vi "Register_Publisher.vi"(11 "Baxter":T3={"topic port"=59814, "Node"="/labview", "topic"="/robot/head/command_head_nod", "type"="std_msgs/Bool", "node port"=7000, "error "={"status"=FALSE, "code"=0, "source"=""}, "Direction"=enum."Publisher", "APIs"=[]}) -> (0 "error out":errorcluster, 2 "connection ID out":refnum<k5>, 3 "Status":T1(ring), 5 "Subscribers":T2(array[cluster]))   [LabVIEW 2013]
doc: "Template server that runs individual ros topics, services, etc. This is cloned for each topic being run."
uses:
  ROS/Code/SubVIs/_ROSControl.ctl
  ROS/Code/SubVIs/_ROSDirection.ctl
  ROS/Code/_ROSDefinition.vi
panel:
  out "tcp":bool
  out "xml":bool
  out "time":u32
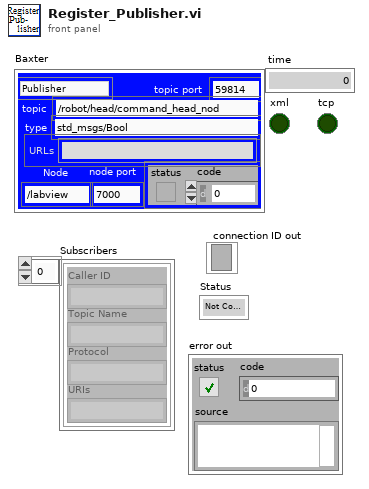
[diagram p1: front panel]
types:
  T1 = enum16{"Not Connected", "Registered", "Connected"}
  T2 = cluster{"Caller ID":string, "Topic Name":string, "Protocol":string, "URIs":string}[]
  T3 = typedef "_ROSControl.ctl" = cluster{"topic port":u16, "Node":string, "topic":string, "type":string, "node port":u32, "error ":errorcluster, "Direction":T4, "APIs":string[]}
  T4 = typedef "_ROSDirection.ctl" = enum16{"Node", "Publisher", "Subscriber", "Service Client"}
  T5 = cluster{"Code":i32, "Status Message":string, "APIs":string[]}
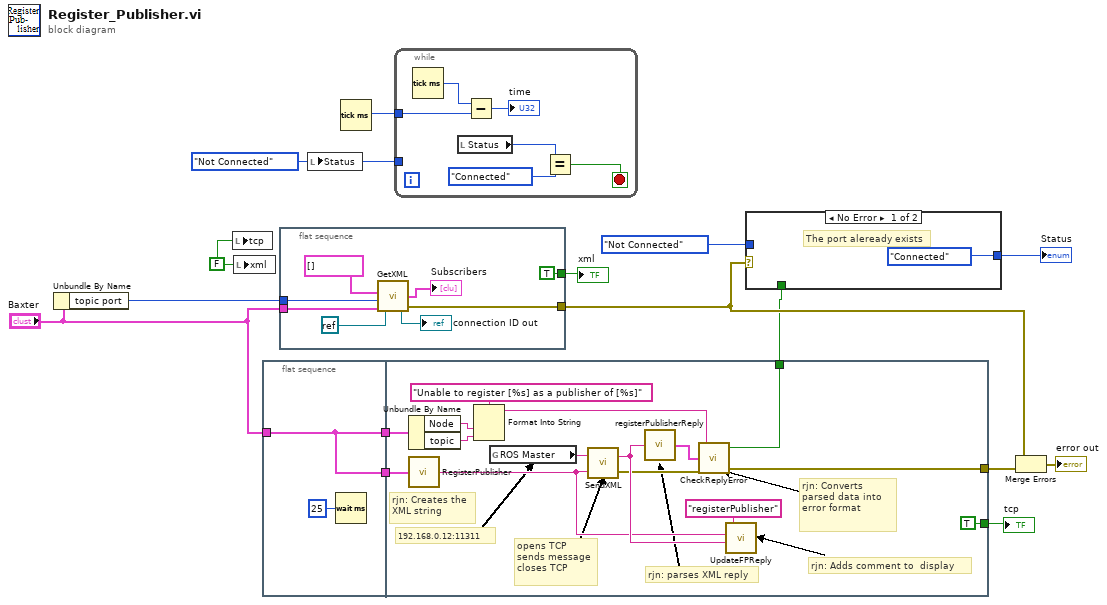
[diagram p0: block diagram]
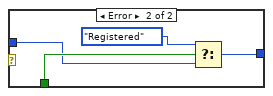
[diagram p2: hidden frame]
diagram:
  w1 = FALSE ("xml")
  w4 = T1."Not Connected" ("Status")
  n1 = Unbundle By Name("Baxter") -> ("topic port"=w15:u16)
  n2 = local write "tcp"(w1) -> ()
  n3 = local write "xml"(w1) -> ()
  n4 = flat-sequence {
    tunnel: "Baxter" -> [w16]
    tunnel: [w16] -> w13
    tunnel: [w16] -> w12
    tunnel: [w22] -> w9
    tunnel: [w20] -> w10
    tunnel: w13 -> [w21]
    tunnel: w12 -> [w19]
    tunnel: [TRUE] -> w2
    frame #0 {
      n5 = Wait (ms)(milliseconds to wait=u32 25) -> ()  [unwired: 1 out]
    }
    frame #1 {
      # "rjn: Adds comment to  display"
      # "rjn: Converts parsed data into\nerror format"
      # "rjn: parses XML reply"
      # "192.168.0.12:11311"
      # "opens TCP\nsends message\ncloses TCP"
      # "rjn: Creates the \nXML string"
      n6 = Unbundle By Name(w21) -> ("Node"=w28:string, "topic"=w27:string)
      n7 = call "RegisterPublisher.vi"("ROS"=w19) -> ("XML"=w26:string)
      n8 = Format Into String(format string="Unable to register [%s] as a publisher of [%s]", w28, w27) -> (resulting string=w24:string)  [unwired: 2 in, 1 out]
      n9 = global read "_ROSDefinition.vi" "ROS Master"() -> (w32:string)
      n10 = call "SendXML.vi"("Send"=w26, "URI in"=w32) -> ("error out"=w23:errorcluster, "Reply"=w31:string)
      n11 = call "registerPublisherReply.vi"("Response"=w31) -> ("Response"=w25:T5)
      n12 = call "CheckReplyError.vi"("error in"=w23, "Response"=w25, "Error String"=w24) -> ("error out"=w20:errorcluster, "Registered?"=w22:bool)  [unwired: 1 out]
      n13 = call "UpdateFPReply.vi"("Reply"=w31, "Sent"=w26, "method"="registerPublisher") -> ()  [unwired: 3 in]
    }
  }
  n14 = flat-sequence {
    tunnel: w15 -> [w40]
    tunnel: "Baxter" -> [w39]
    tunnel: [w38] -> w11
    tunnel: [TRUE] -> w3
    frame #0 {
      n15 = call "GetXML.vi"("Baxter"=w39, "topic port"=w40, "Connections"=T2 [], "connection ID in"=refnum<k0> refnum) -> ("error IO"=w38:errorcluster, "Subscribers"=→"Subscribers":T2, "connection ID out"=→"connection ID out":refnum<k5>)
    }
  }
  n16 = local write "Status"(w4) -> ()
  n17 = Tick Count (ms)() -> (millisecond timer value=w5:u32)
  n18 = while {
    tunnel: w5 -> [w45]
    tunnel: w4 -> [_]
    stop <- w41 stop-if-true
    n19 = Tick Count (ms)() -> (millisecond timer value=w46:u32)
    n20 = local read "Status"() -> (w43:T1)
    n21 = Subtract(x=w46, y=w45) -> (x-y=→"time":u32)
    n22 = Equal?(x=w43, y=T1."Connected" ("f")) -> (x = y?=w41:bool)
  }
  n23 = case shown="No Error" w11 {
    tunnel: w9 -> [_ w51]
    tunnel: T1."Not Connected" ("Status") -> [_ w50]
    tunnel: [T1."Connected" ("f") w48] -> w8
    frame No Error {
      # "The port aleready exists"
    }
    frame Error {
      n24 = Select(t=T1."Registered", s=w51, f=w50) -> (s? t:f=w48:T1)
    }
  }
  "Status" <- w8
  n25 = Merge Errors(w11, w10) -> (→"error out":errorcluster)
  "xml" <- w3
  "tcp" <- w2
